vi "PicoScope4000aNearestSampleInterval.vi"(5 "Enabled array":i16[](array[numeric])=[0, 0, 0, 0, 0, 0, 0, 0, 0, 0], 6 "Acquisition Settings":T1 {"postTriggerSamples" format="%_6p"; "preTriggerSamples" format="%_6p"}, 7 "Resolution":u32(ring)=10 items=["8-bit"=0, "12-bit"=1, "14-bit"=2, "15-bit"=3, "16-bit"=4, "10-bit"=10], 8 "error in (no error)":errorcluster, 9 "roundFaster":bool, 10 "timeIntervalRequested":dbl format="%#6_6p", 11 "handle in":i16) -> (0 "error out":errorcluster, 1 "timebase":u32, 2 "timeIntervalAvailable":dbl format="%#6_6p", 3 "handle out":i16)   [LabVIEW 2010]
doc: "Calls Gettimebase function"
uses:
  ps4000a.dll
  shared/Acquisition Settings.ctl
panel:
  in  "Memory Segment":u32
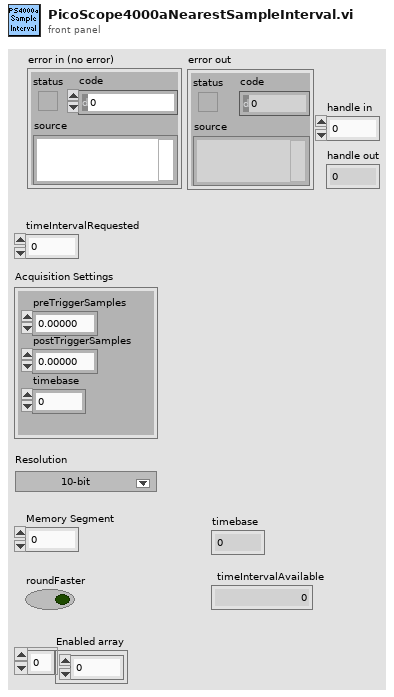
[diagram p1: front panel]
types:
  T1 = typedef "Acquisition Settings.ctl" = cluster{"preTriggerSamples":u64, "postTriggerSamples":u64, "timebase":u32}
  T2 = cluster{"status":bool, "code":u32, "source":string}
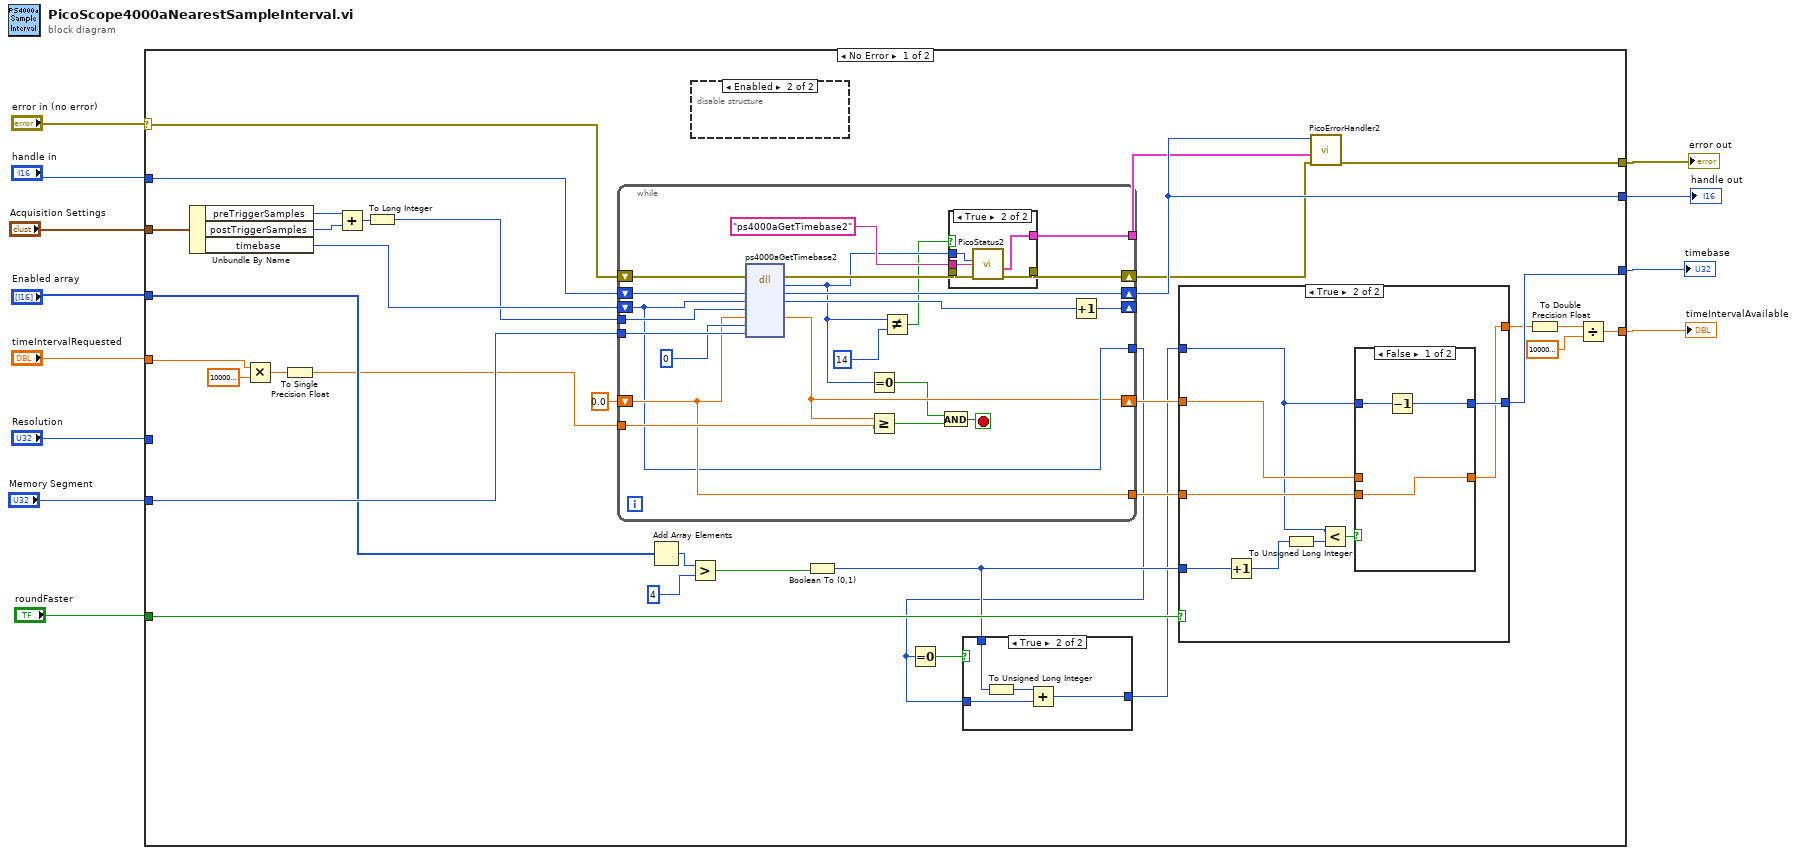
[diagram p0: block diagram]
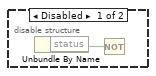
[diagram p2: hidden frame]
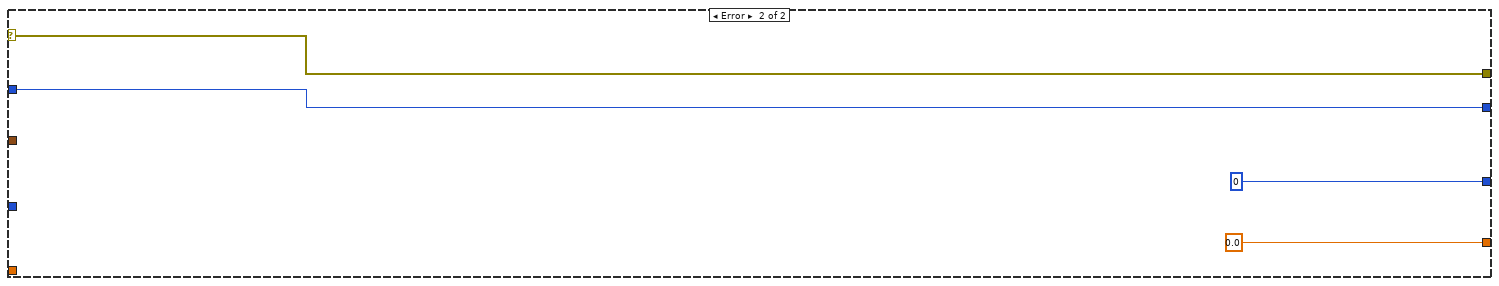
[diagram p7: hidden frame]
diagram:
  n1 = case shown="No Error" "error in (no error)" {
    selector: "error in (no error)" -> [w19 w100]
    tunnel: [w46 w100] -> w12
    tunnel: [w37 w99] -> w11
    tunnel: "handle in" -> [w38 w99]
    tunnel: "Enabled array" -> [w24 _]
    tunnel: "Resolution" -> [_ _]
    tunnel: "roundFaster" -> [w30 _]
    tunnel: "timeIntervalRequested" -> [w43 _]
    tunnel: [w27 u32 0 ("timebase")] -> w4
    tunnel: [w34 0.0 ("timeIntervalAvailable")] -> w3
    tunnel: "Acquisition Settings" -> [w39 _]
    tunnel: "Memory Segment" -> [w36 _]
    frame No Error {
      n2 = Unbundle By Name(w39) -> ("preTriggerSamples"=w41:u64, "postTriggerSamples"=w42:u64, "timebase"=w31:u32)
      n3 = Multiply(x=w43, y=1000000000.0) -> (x*y=w44:dbl)
      n4 = To Single Precision Float(number=w44) -> (single precision float=w17:sgl)
      n5 = Add(x=w41, y=w42) -> (x+y=w40:u64)
      n6 = To Long Integer(number=w40) -> (32bit integer=w20:i32)
      n7 = while {
        tunnel: w20 -> [w90]
        tunnel: w36 -> [w87]
        shift-right: [w88] -> w37
        shift-left: w38 -> [w89]
        shift-right: [w84] -> w33
        shift-left: w19 -> [w72]
        tunnel: [w82] -> w32
        shift-right: [w81] -> _
        shift-left: w31 -> [w77]
        tunnel: w17 -> [w80]
        shift-right: [w76] -> w28
        shift-left: sgl 0.0 ("timeIntervalNanoseconds") -> [w78]
        tunnel: [w78] -> w29
        tunnel: [w77] -> w18
        stop <- w75 stop-if-true
        n8 = dll-call lib="ps4000a.dll" fn="ps4000aGetTimebase2"(error in=w72, "handle"=w89, "timebase"=w77, "noSamples"=w90, "timeIntervalNanoseconds"=w78, "maxSamples"=0, "segmentIndex"=w87) -> (error out=w85:errorcluster, "PICO_STATUS"=w71:u32, "handle"=w88:i16, "timebase"=w79:u32, "timeIntervalNanoseconds"=w76:sgl)  [unwired: 5 in, 1 out]
        n9 = Equal To 0?(x=w71) -> (x = 0?=w73:bool)
        n10 = Greater Or Equal?(x=w76, y=w80) -> (x >= y?=w74:bool)
        n11 = Not Equal?(x=w71, y=u32 14) -> (x != y?=w69:bool)
        n12 = And(x=w73, y=w74) -> (x .and. y?=w75:bool)
        n13 = case shown="True" w69 {
          tunnel: w85 -> [w91 w96]
          tunnel: [w91 w95] -> w84
          tunnel: "ps4000aGetTimebase2" ("source") -> [_ w94]
          tunnel: [_ w93] -> w82
          tunnel: w71 -> [_ w92]
          frame False {
          }
          frame True {
            n14 = call "PicoStatus2.vi"("PICO source"=w94, "Error in"=w96, "PICO STATUS"=w92) -> ("error out"=w95:errorcluster, "PICO_STATUS out"=w93:T2)  [unwired: 5 in]
          }
        }
        n15 = Increment(x=w79) -> (x+1=w81:u32)
      }
      n16 = Add Array Elements(numeric array=w24) -> (sum=w25:i16)
      n17 = Greater?(x=w25, y=i16 4) -> (0:w23:bool)
      n18 = disable-structure shown="Enabled" {
        frame Disabled {
          n19 = Unbundle By Name() -> ("status"=w47:bool)  [unwired: 1 in]
          n20 = Not(x=w47) -> ()  [unwired: 1 out]
        }
        frame Enabled {
        }
      }
      n21 = Boolean To (0,1)(Boolean=w23) -> (0, 1=w21:i16)
      n22 = Equal To 0?(x=w18) -> (x = 0?=w22:bool)
      n23 = case shown="True" w22 {
        tunnel: w18 -> [w48 w52]
        tunnel: w21 -> [_ w49]
        tunnel: [w48 w51] -> w15
        frame False {
        }
        frame True {
          n24 = To Unsigned Long Integer(number=w49) -> (unsigned 32bit integer=w50:u32)
          n25 = Add(x=w50, y=w52) -> (x+y=w51:u32)
        }
      }
      n26 = case shown="True" w30 {
        tunnel: [w54 w62] -> w13
        tunnel: w29 -> [_ w61]
        tunnel: w28 -> [w54 w60]
        tunnel: [w53 w63] -> w27
        tunnel: w15 -> [w53 w57]
        tunnel: w21 -> [_ w58]
        frame False {
        }
        frame True {
          n27 = Increment(x=w58) -> (x+1=w56:i16)
          n28 = To Unsigned Long Integer(number=w56) -> (unsigned 32bit integer=w55:u32)
          n29 = Less?(x=w57, y=w55) -> (x < y?=w59:bool)
          n30 = case shown="False" w59 {
            tunnel: [w66 w68] -> w63
            tunnel: w57 -> [w65 w68]
            tunnel: [w64 w67] -> w62
            tunnel: w61 -> [w64 _]
            tunnel: w60 -> [_ w67]
            frame False {
              n31 = Decrement(x=w65) -> (x-1=w66:u32)
            }
            frame True {
            }
          }
        }
      }
      n32 = call "PicoErrorHandler2.vi"("error in (no error)"=w33, "PICO_STATUS in"=w32, "handle In"=w37) -> ("error out"=w46:errorcluster)  [unwired: 8 in]
      n33 = To Double Precision Float(number=w13) -> (double precision float=w14:dbl)
      n34 = Divide(x=w14, y=1000000000.0) -> (x/y=w34:dbl)
    }
    frame Error {
    }
  }
  "error out" <- w12
  "handle out" <- w11
  "timebase" <- w4
  "timeIntervalAvailable" <- w3
